vi "Ok Prompt.vi"(8 "error in":errorcluster, 11 "Message":string) -> (0 "error out":errorcluster)   [LabVIEW 2018]
panel:
  in  "OK Button":bool
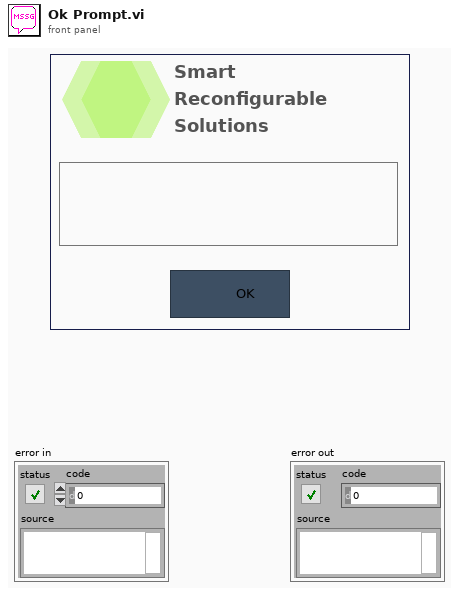
[diagram p1: front panel]
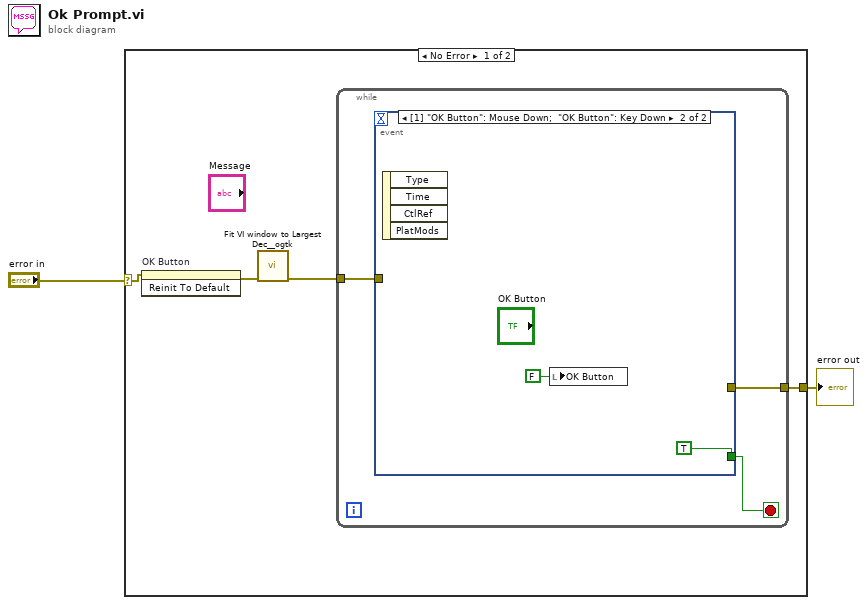
[diagram p0: block diagram]
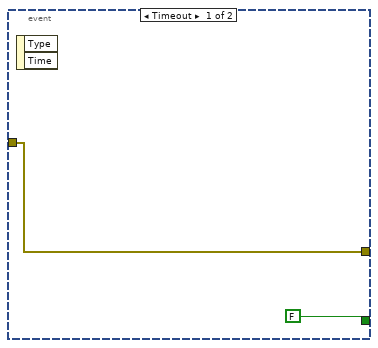
[diagram p2: hidden frame]
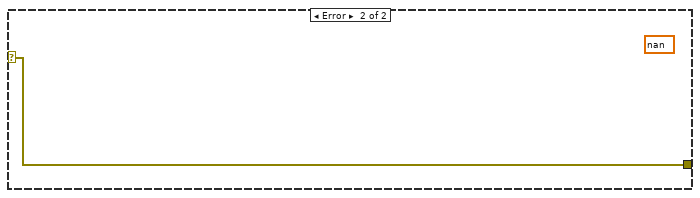
[diagram p3: hidden frame]
diagram:
  n1 = case shown="No Error" "error in" {
    selector: "error in" -> [w4 w14]
    tunnel: [w5 w14] -> w1
    frame No Error {
      n2 = invoke on="OK Button" class="Bool (strict)" method="Reinit To Default"(error in=w4) -> (error out=w6:errorcluster)  [unwired: 2 in, 2 out]
      n3 = call <userlib>:"Fit VI window to Largest Dec__ogtk.vi"("error in (no error)"=w6) -> ("error out"=w3:errorcluster)  [unwired: 5 in, 1 out]
      n4 = while {
        tunnel: w3 -> [w9]
        tunnel: [w8] -> w5
        stop <- w7 stop-if-true
        n5 = event shown="[1] \"OK Button\": Mouse Down;  \"OK Button\": Key Down" {
          selector: _ -> [_ _]
          dyn-events: _ -> [_ _]
          timeout: _ -> [_ _]
          tunnel: w9 -> [w11 _]
          tunnel: [w11 _] -> w8
          tunnel: [FALSE TRUE] -> w7
          event Timeout {
            n6 = event-data() -> ()  [unwired: 1 in, 2 out]
          }
          event "OK Button": Mouse Down; "OK Button": Key Down {
            n7 = event-data() -> ()  [unwired: 1 in, 4 out]
            n8 = local write "OK Button"(FALSE ("OK Button")) -> ()
          }
        }
      }
    }
    frame Error {
      (unwired) nan ("Numeric Control")
    }
  }
  "error out" <- w1
